vi "SET - Triggered Events & Data.vi"(8 "error in (no error)":errorcluster, 9 "Data":string="Hi!!!", 10 "Events":T1, 11 "Parent_Class in":refnum<class "Message_Distributor_Class.lvclass">) -> (0 "error out":errorcluster, 3 "Parent_Class out":refnum<class "Message_Distributor_Class.lvclass">)   [LabVIEW 2023, in "Actor_Message_Distributor.lvlib" / "Message_Distributor_Class.lvclass"]
uses:
  Message_Distributor_Class.lvclass
  Abstraction_Interface_Class/Usr Ev/Ctrl - Enum - Events.ctl
  Message_Distributor_Class.lvclass/Message_Distributor_Class.ctl
  Abstraction_Interface_Class/Abstraction_Interface_Class.lvclass
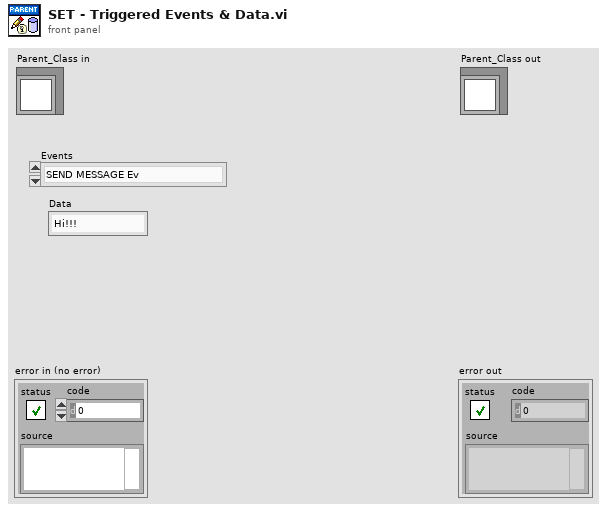
[diagram p1: front panel]
types:
  T1 = typedef "Abstraction_Interface.lvlib/Abstraction_Interface_Class.lvclass/Ctrl - Enum - Events.ctl" = enum16{"SEND MESSAGE Ev", "STOP_ACTOR Ev", "INIT_ACTOR Ev", "START Ev", "STOP Ev", "GET Ev", "SET Ev", "ERROR_HANDLER Ev", "RESET Ev"}
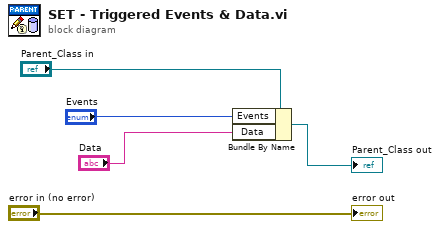
[diagram p0: block diagram]
diagram:
  n1 = Bundle By Name(cluster="Parent_Class in", "Events"="Events", "Data"="Data") -> (→"Parent_Class out":refnum<class "Message_Distributor_Class.lvclass">)
  "error out" <- "error in (no error)"
